vi "Reset.vi"(8 "error in (no error)":errorcluster, 11 "Proto Tag in":refnum<class "Raw Message.lvclass">) -> (0 "error out":errorcluster, 3 "Proto Tag out":refnum<class "Raw Message.lvclass">)   [LabVIEW 2020, in "Protobuf RAW.lvlib" / "Raw Message.lvclass"]
uses:
  Raw Message.lvclass
  Raw Message.lvclass/Raw Message.ctl
  Tag/Basic Type.lvclass
  Proto Type Common/Proto Type Common.lvclass
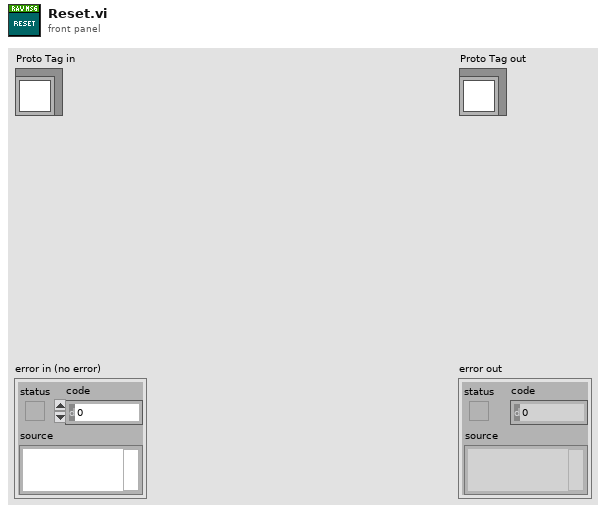
[diagram p1: front panel]
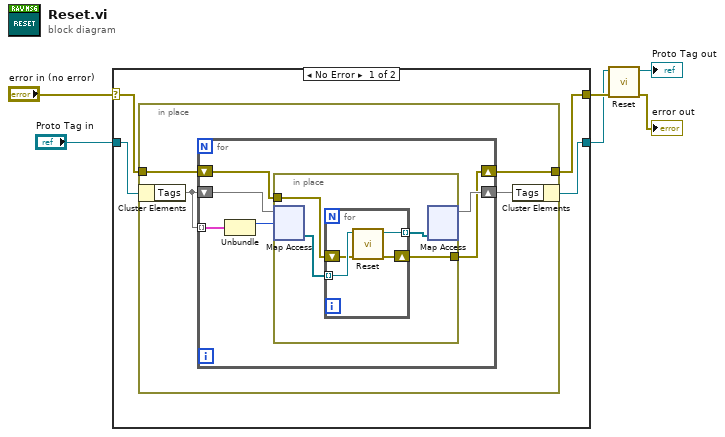
[diagram p0: block diagram]
diagram:
  n1 = case shown="No Error" "error in (no error)" {
    selector: "error in (no error)" -> [w8 w29]
    tunnel: "Proto Tag in" -> [w10 w30]
    tunnel: [w9 w30] -> w2
    tunnel: [w7 w29] -> w4
    frame No Error {
      n2 = in-place {
        in-place-border: w8 -> [w12]
        in-place-border: [w11] -> w7
        n3 = in-place-cluster #1(w10) -> ("Tags"=w13:map{u32, refnum<class "Basic Type.lvclass">[]})
        n4 = for {
          shift-right: [w19] -> w14
          shift-left: w13 -> [w20]
          tunnel: w13 -> [w18] mode=indexing
          shift-right: [w15] -> w11
          shift-left: w12 -> [w16]
          n5 = Unbundle(w18) -> ("ID"=w17:u32)  [unwired: 1 out]
          n6 = in-place {
            in-place-border: w16 -> [w22]
            in-place-border: [w21] -> w15
            n7 = in-place-map #2(w20, w17) -> (w24:refnum<class "Basic Type.lvclass">[])  [unwired: 1 in, 1 out]
            n8 = for {
              tunnel: w24 -> [w28] mode=indexing
              tunnel: [w27] -> w23 mode=indexing
              shift-right: [w25] -> w21
              shift-left: w22 -> [w26]
              n9 = call-dynamic "Reset.vi"("error in (no error)"=w26, "Proto Tag in"=w28) -> ("error out"=w25:errorcluster, "Proto Tag out"=w27:refnum<class "Basic Type.lvclass">)  [unwired: 8 in]
            }
            n10 = in-place-map #2(w23) -> (w19:map{u32, refnum<class "Basic Type.lvclass">[]})  [unwired: 1 in, 2 out]
          }
        }
        n11 = in-place-cluster #1("Tags"=w14) -> (w9:refnum<class "Raw Message.lvclass">)
      }
    }
    frame Error {
    }
  }
  n12 = call-parent "Reset.vi"("error in (no error)"=w4, "Proto Type Common in"=w2) -> ("error out"=→"error out":errorcluster, "Proto Type Common out"=→"Proto Tag out":refnum<class "Raw Message.lvclass">)  [unwired: 8 in]
